vi "Get Status Channels for Tx Message.vi"(8 "error in":errorcluster, 11 "message in":T1 format="%.0x") -> (0 "error out":errorcluster, 2 "status channels":T1[](array[typedef]) format="%.0x", 3 "message out":T1 format="%.0x", 4 "found?":bool)   [LabVIEW 2020, in "Ballard MIL-STD-1553 Scripting.lvlib"]
uses:
  Ballard MIL-STD-1553 Scripting.lvlib
  <vilib>/NI VeriStand/Custom Device Tools/Custom Device Utility Library/Custom Device Utility Library.lvlib
  Constants.vi
  <vilib>/NI VeriStand/Custom Device Tools/Custom Device Utility Library/Search Direction.ctl
  <vilib>/NI VeriStand/Custom Device Tools/Custom Device Utility Library/NI VeriStand - Search for Item by GUID.vi
  <vilib>/NI VeriStand/Custom Device API/Custom Device Item Ref.ctl
  <vilib>/NI VeriStand/Custom Device API/Custom Device API.lvlib
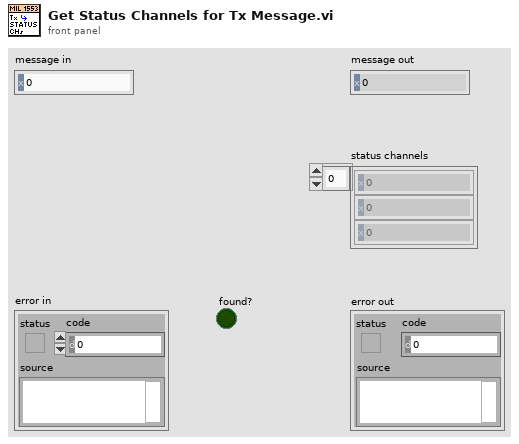
[diagram p1: front panel]
types:
  T1 = typedef "Custom Device API.lvlib/Custom Device Item Ref.ctl" = u64
  T2 = typedef "Custom Device Utility Library.lvlib/Search Direction.ctl" = enum16{"Down", "Up"}
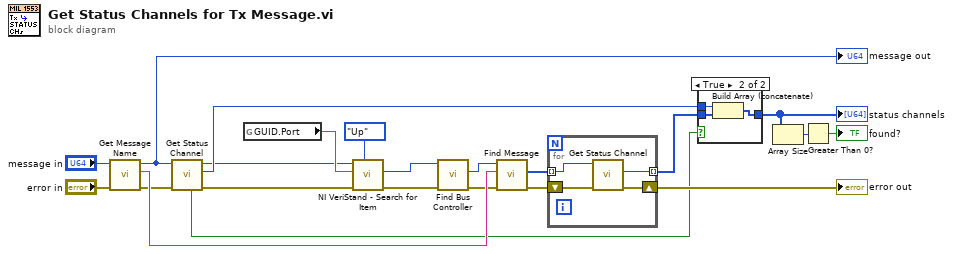
[diagram p0: block diagram]
diagram:
  n1 = call "Get Message Name.vi"("error in"="error in", "message in"="message in") -> ("error out"=w7:errorcluster, "message name"=w17:string, "message out"=w2:T1)  [unwired: 6 in, 1 out]
  "message out" <- w2
  n2 = call "Get Status Channel.vi"("error in"=w7, "section reference in"=w2) -> ("error out"=w8:errorcluster, "status channel"=w15:T1, "section reference out"=w9:T1, "found?"=w1:bool)  [unwired: 6 in]
  n3 = global read "Constants.vi" "GUID.Port"() -> (w22:string)
  n4 = call-poly <vilib>:"NI VeriStand - Search for Item.vi"("Direction (Down)"=Search_Direction."Up", "error in"=w8, "Item GUID"=w22, "Section Ref in"=w9) -> ("error out"=w19:errorcluster, "Item Ref"=w20:T1)  [unwired: 4 in, 2 out]
  n5 = call "Find Bus Controller.vi"("error in"=w19, "port in"=w20) -> ("error out"=w16:errorcluster, "bus controller"=w18:T1)  [unwired: 6 in, 2 out]
  n6 = call "Find Message.vi"("error in"=w16, "message name"=w17, "port in"=w18) -> ("error out"=w6:errorcluster, "message refs"=w5:T1[])  [unwired: 5 in, 2 out]
  n7 = for {
    tunnel: w5 -> [w25] mode=indexing
    shift-right: [w24] -> w4
    shift-left: w6 -> [w26]
    tunnel: [w23] -> w3 mode=indexing
    n8 = call "Get Status Channel.vi"("error in"=w26, "section reference in"=w25) -> ("error out"=w24:errorcluster, "status channel"=w23:T1)  [unwired: 6 in, 2 out]
  }
  "error out" <- w4
  n9 = case shown="True" w1 {
    tunnel: w15 -> [_ w30]
    tunnel: [w27 w29] -> w13
    tunnel: w3 -> [w27 w28]
    frame False {
    }
    frame True {
      n10 = Build Array (concatenate)(w30, w28) -> (w29:T1[])
    }
  }
  "status channels" <- w13
  n11 = Array Size(array=w13) -> (size(s)=w14:i32)
  n12 = Greater Than 0?(x=w14) -> (x > 0?=→"found?":bool)
